vi "Write elVelocity.vi"(8 "error in (no error)":errorcluster, 10 "elVelocity":dbl[unit] min=-0.3490658503988659 max=0.3490658503988659, 11 "AzElTracking in":refnum<class "AzElTracking.lvclass">) -> (0 "error out":errorcluster, 3 "AzElTracking out":refnum<class "AzElTracking.lvclass">)   [LabVIEW 2022 SP3, in "TCSDataDefinitions.lvlib" / "TCSMountControlStatus.lvlib" / "AzElTracking.lvclass"]
uses:
  AzElTracking.lvclass
  AzElTracking.lvclass/AzElTracking.ctl
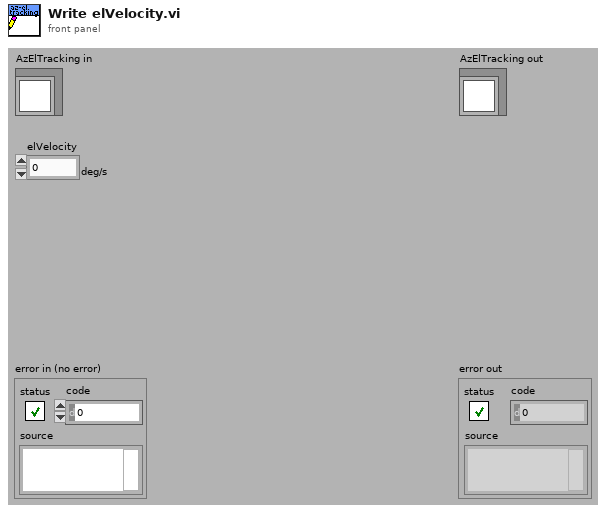
[diagram p1: front panel]
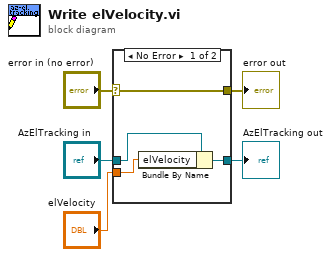
[diagram p0: block diagram]
diagram:
  n1 = case shown="No Error" "error in (no error)" {
    selector: "error in (no error)" -> [w9 w10]
    tunnel: [w9 w10] -> w4
    tunnel: [w7 w11] -> w2
    tunnel: "AzElTracking in" -> [w8 w11]
    tunnel: "elVelocity" -> [w6 _]
    frame No Error {
      n2 = Bundle By Name(cluster=w8, "elVelocity"=w6) -> (w7:refnum<class "AzElTracking.lvclass">)
    }
    frame Error {
    }
  }
  "error out" <- w4
  "AzElTracking out" <- w2
